vi "SFOAE-Append Raw Data.vi"(0 "DataProc In":T1, 7 "Buffer":dbl[](array[numeric]), 11 "error in (no error)":errorcluster) -> (4 "DataProc Out":T1, 15 "error out":errorcluster)   [LabVIEW 2020]
uses:
  Typedefs/SFOAE-Data Processing.ctl
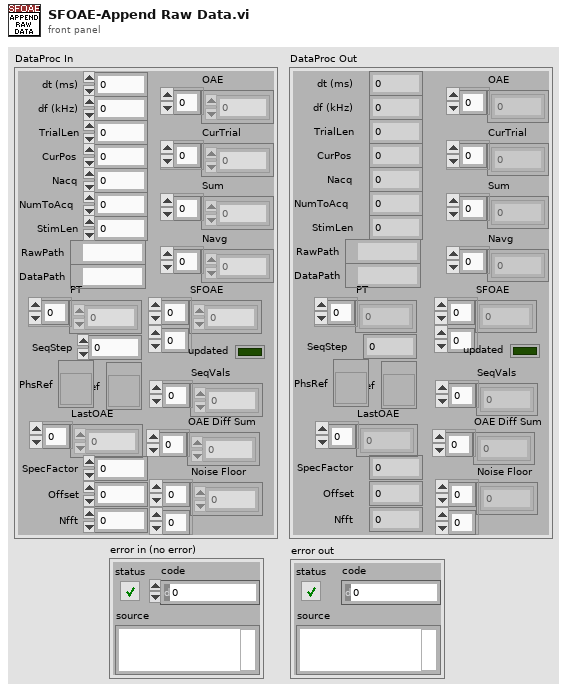
[diagram p1: front panel]
types:
  T1 = typedef "SFOAE-Data Processing.ctl" = cluster{"dt (ms)":dbl, "TrialLen":i32, "PT":cdb[], "CurPos":i32, "Sum":dbl[], "Navg":dbl[], "Nacq":i32, "RawPath":path, "DataPath":path, "NumToAcq":i32, "OAE":dbl[], "CurTrial":dbl[], "StimLen":i32, "SFOAE":cdb[][], "SeqStep":i32, "updated":bool, "SeqVals":dbl[], "df (kHz)":dbl, "MagRef":refnum<vi>, "LastOAE":dbl[], "OAE Diff Sum":dbl[], "Noise Floor":cdb[][], "SpecFactor":dbl, "Offset":i32, "Nfft":i32, "PhsRef":refnum<vi>}
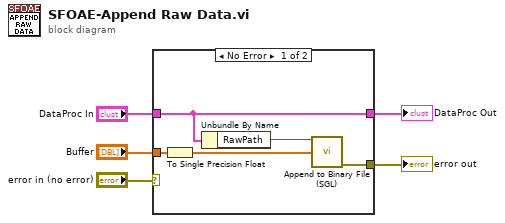
[diagram p0: block diagram]
diagram:
  n1 = case shown="No Error" "error in (no error)" {
    selector: "error in (no error)" -> [_ w11]
    tunnel: "DataProc In" -> [w10 w12]
    tunnel: [w10 w12] -> w2
    tunnel: [w8 w11] -> w4
    tunnel: "Buffer" -> [w7 _]
    frame No Error {
      n2 = To Single Precision Float(number=w7) -> (single precision float=w6:sgl[])
      n3 = Unbundle By Name(w10) -> ("RawPath"=w9:path)
      n4 = call "Append to Binary File (SGL).vi"("file path"=w9, "data"=w6) -> ("error out"=w8:errorcluster)  [unwired: 12 in, 1 out]
    }
    frame Error {
    }
  }
  "error out" <- w4
  "DataProc Out" <- w2
